vi "Reorganize&ScaleMeasurements.vi"(4 "dt":dbl=0.1 format="%#_13g", 6 "error-status":u8, 7 "MeasurementType":string, 8 "Error In":errorcluster, 9 "Error String":string, 10 "SNMPDataAsStrings":string[](array[string])) -> (0 "Error Out":errorcluster, 1 "Numerical Information":bool, 2 "String":string, 3 "output waveform":waveform(dbl))   [LabVIEW 2018, in "SensorPlugins.lvlib" / "RoomAlert.lvclass"]
uses:
  RoomAlert.lvclass
panel:
  out "replaced":bool
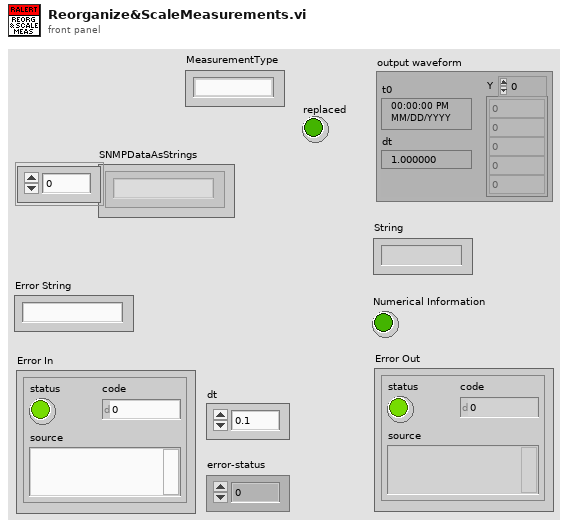
[diagram p1: front panel]
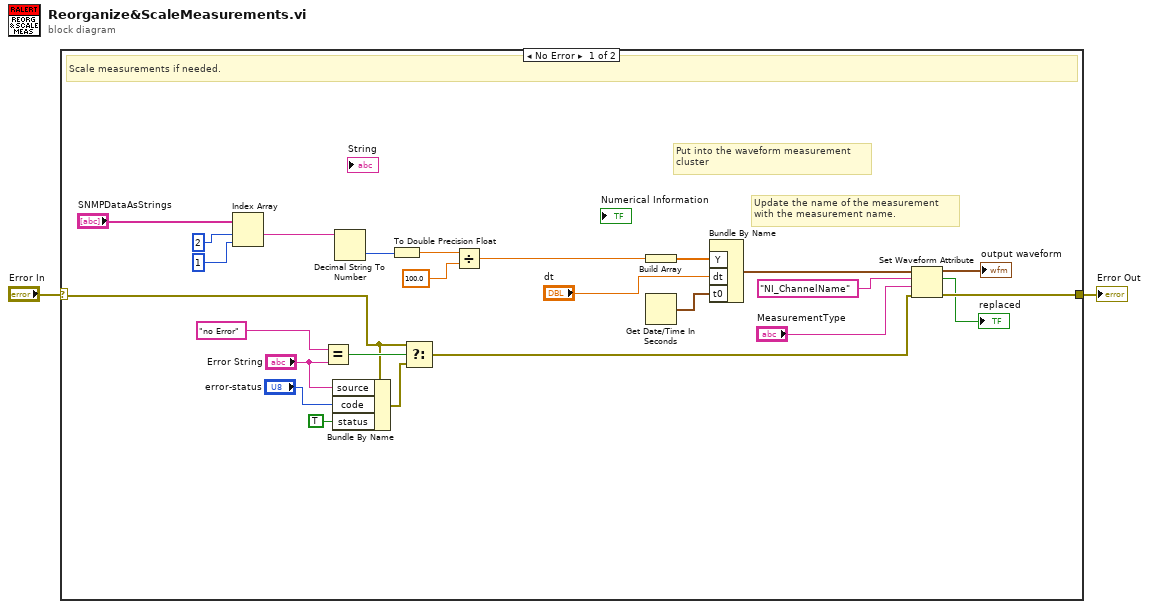
[diagram p0: block diagram]
diagram:
  n1 = case shown="No Error" "Error In" {
    selector: "Error In" -> [w16 w28]
    tunnel: [w23 w28] -> w2
    frame No Error {
      # "Update the name of the measurement \nwith the measurement name."
      # "Put into the waveform measurement\ncluster"
      # "Scale measurements if needed."
      n2 = Index Array(array="SNMPDataAsStrings", index #1=2 ("disabled index (col)"), index #2=1 ("index (col)")) -> (element #1=w10:string)  [unwired: 1 out]
      n3 = Equal?(x="no Error" ("error-string"), y="Error String") -> (x = y?=w17:bool)
      n4 = Bundle By Name(cluster=w16, "source"="Error String", "code"="error-status", "status"=TRUE) -> (w11:errorcluster)
      n5 = Decimal String To Number(string=w10) -> (number=w4:i32)  [unwired: 2 in, 1 out]
      n6 = To Double Precision Float(number=w4) -> (double precision float=w3:dbl)
      n7 = Select(t=w16, s=w17, f=w11) -> (s? t:f=w12:errorcluster)
      n8 = Divide(x=w3, y=100.0 ("SNMPDataAsStrings")) -> (x/y=w6:dbl)
      n9 = Build Array(w6) -> (w5:dbl[])
      n10 = Get Date/Time In Seconds() -> (seconds since 1Jan1904=w27:timestamp)
      n11 = Bundle By Name("Y"=w5, "dt"="dt", "t0"=w27) -> (w25:waveform(dbl))  [unwired: 1 in]
      n12 = Set Waveform Attribute(4:w12, 5:"MeasurementType", 6:"NI_ChannelName" ("name"), 7:w25) -> (0:w23:errorcluster, 2:→"replaced":bool, 3:→"output waveform":waveform(dbl))
    }
    frame Error {
    }
  }
  "Error Out" <- w2
